vi "System info.vi"() -> ()   [LabVIEW 2016]
panel:
  in  "Max coinchunt lim":i32=900
  in  "TDCRead Buffer Size":i32=3300
  in  "# of threads":i32=4
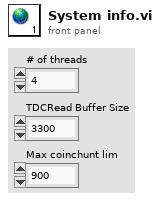
[diagram p1: front panel]
diagram:
